vi "NotifyIcon - Create Menu.vi"(8 "error in":errorcluster, 9 "lookup string":string, 11 "Menus":string[][](array[string])=[["item0", "<submenu0>"], ["item1", "submenuitem0"], ["<submenu0>", ""]]) -> (0 "error out":errorcluster, 2 "MenuItem references":refnum<k24>[](array[refnum]))   [LabVIEW 2020]
doc: "Recursive"
uses:
  System.Windows.Forms
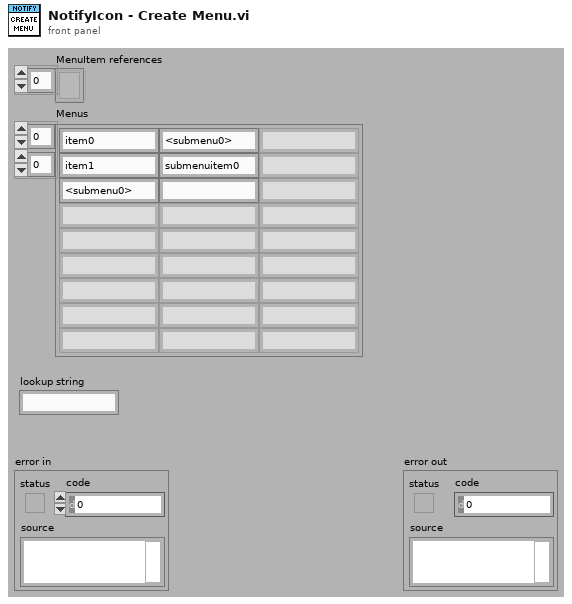
[diagram p1: front panel]
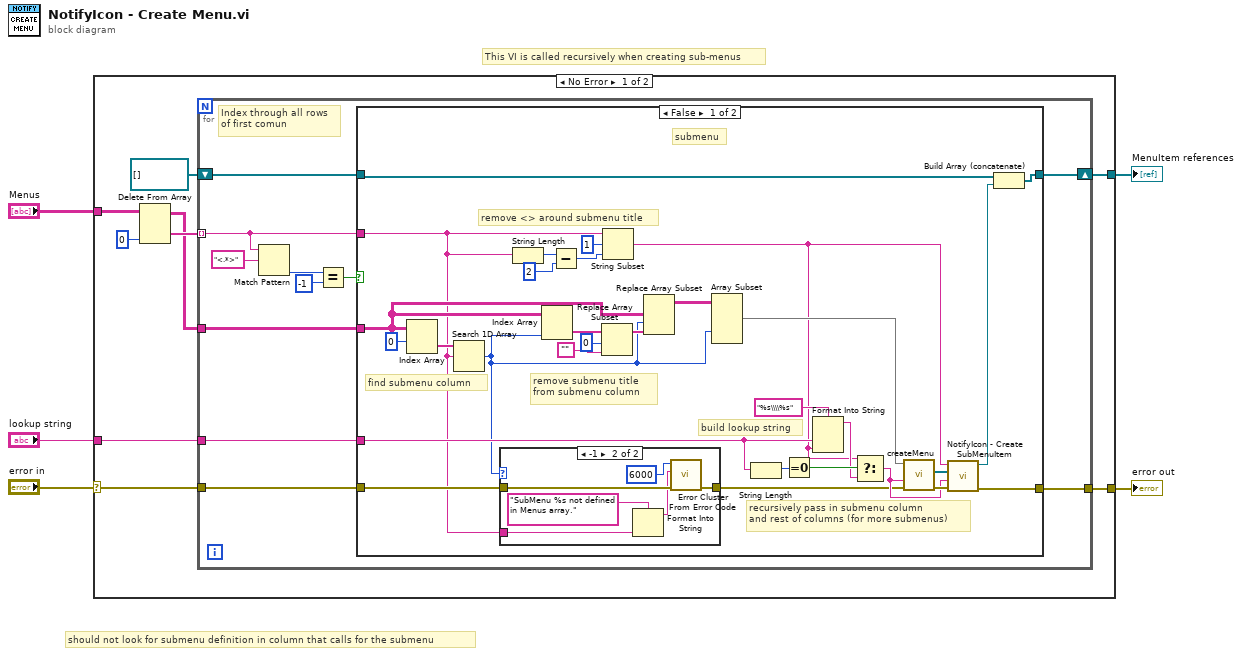
[diagram p0: block diagram]
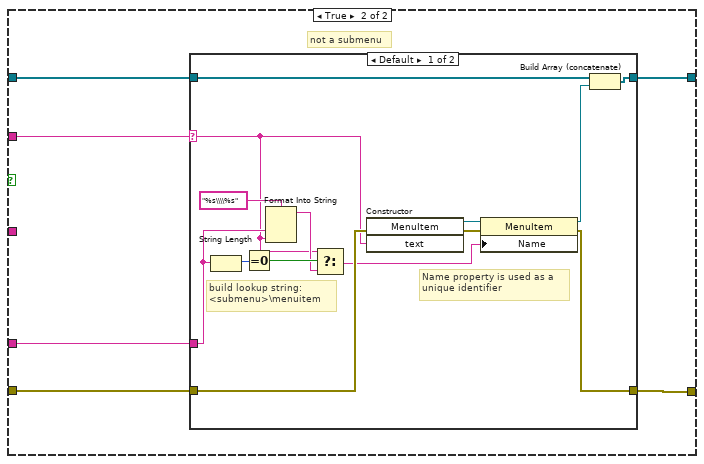
[diagram p3: hidden frame]
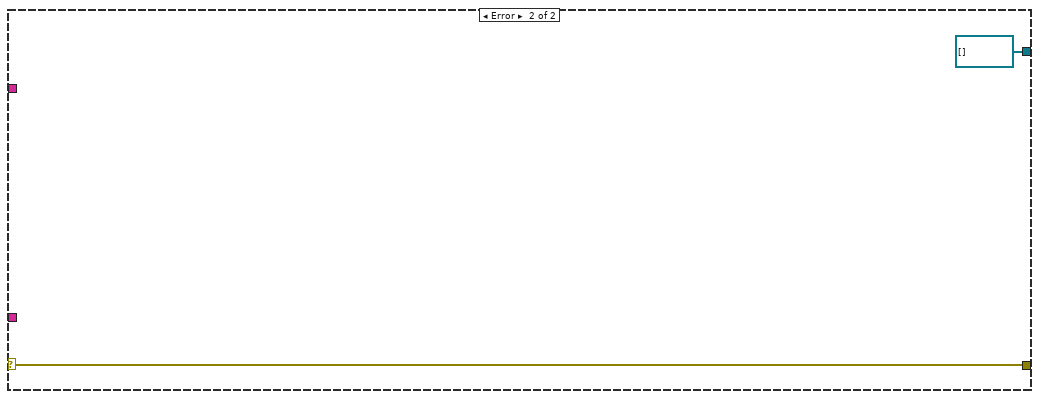
[diagram p5: hidden frame]
diagram:
  # "should not look for submenu definition in column that calls for the submenu"
  # "This VI is called recursively when creating sub-menus"
  n1 = case shown="No Error" "error in" {
    selector: "error in" -> [w10 w86]
    tunnel: [w14 refnum<k24>[] []] -> w5
    tunnel: "Menus" -> [w9 _]
    tunnel: [w12 w86] -> w3
    tunnel: "lookup string" -> [w11 _]
    frame No Error {
      n2 = Delete From Array(array=w9, index (col)=0 ("disabled index (col)")) -> (deleted portion=w7:string[], array with subset deleted=w6:string[][])  [unwired: 2 in]
      n3 = for {
        tunnel: w7 -> [w21] mode=indexing
        shift-right: [w20] -> w14
        shift-left: refnum<k24>[] [] -> [w19]
        tunnel: w6 -> [w18]
        tunnel: w10 -> [w17]
        tunnel: [w16] -> w12
        tunnel: w11 -> [w15]
        # "Index through all rows\nof first comun"
        n4 = Match Pattern(string=w21, regular expression="<.*>") -> (offset past match=w24:i32)  [unwired: 1 in, 3 out]
        n5 = Equal?(x=w24, y=-1) -> (x = y?=w22:bool)
        n6 = case shown="False" w22 {
          tunnel: w21 -> [w26 w64]
          tunnel: [w49 w68] -> w20
          tunnel: w19 -> [w48 w67]
          tunnel: w18 -> [w44 _]
          tunnel: w17 -> [w28 w66]
          tunnel: [w40 w65] -> w16
          tunnel: w15 -> [w35 w63]
          frame False {
            # "build lookup string"
            # "recursively pass in submenu column\nand rest of columns (for more submenus)"
            # "remove submenu title\nfrom submenu column"
            # "find submenu column"
            # "remove <> around submenu title"
            # "submenu"
            n7 = Index Array(array=w44, index (row)=0) -> (element=w50:string[])  [unwired: 1 in]
            n8 = Search 1D Array(1D array=w50, element=w26) -> (index of element=w29:i32)  [unwired: 1 in]
            n9 = case shown="-1" w29 {
              tunnel: w28 -> [w56 w62]
              tunnel: [w56 w61] -> w27
              tunnel: w26 -> [_ w59]
              frame 0, Default {
              }
              frame -1 {
                n10 = Format Into String(format string="SubMenu %s not defined in Menus array." ("error message (\"\")"), w59) -> (resulting string=w58:string)  [unwired: 2 in, 1 out]
                n11 = call <vilib>:"Error Cluster From Error Code.vi"("error in (no error)"=w62, "error message (\"\")"=w58, "error code (0)"=6000) -> ("error out"=w61:errorcluster)  [unwired: 6 in]
              }
            }
            n12 = String Length(string=w26) -> (length=w53:i32)
            n13 = Index Array(array=w44, index (col)=w29) -> (element=w45:string[])  [unwired: 1 in]
            n14 = Subtract(x=w53, y=2) -> (x-y=w51:i32)
            n15 = Replace Array Subset(array=w45, new element="", index=0) -> (w43:string[])
            n16 = String Subset(string=w26, offset (0)=1, length (rest)=w51) -> (substring=w31:string)
            n17 = Replace Array Subset(array=w44, new element=w43, index (col)=w29) -> (w42:string[][])  [unwired: 1 in]
            n18 = Array Subset(array=w42, index (col)=w29) -> (w37:string[][])  [unwired: 3 in]
            n19 = String Length(string=w35) -> (length=w34:i32)
            n20 = Equal To 0?(x=w34) -> (x = 0?=w33:bool)
            n21 = Format Into String(format string="%s\\\\%s", w35, w31) -> (resulting string=w32:string)  [unwired: 2 in, 1 out]
            n22 = Select(t=w31, s=w33, f=w32) -> (s? t:f=w30:string)
            n23 = call "createMenu.vi"("error in"=w27, "lookup string"=w30, "Menus"=w37) -> ("error out"=w39:errorcluster, "MenuItem references"=w46:refnum<k24>[])  [unwired: 7 in]
            n24 = call "NotifyIcon - Create SubMenuItem.vi"("error in"=w39, "lookup string"=w30, "MenuItem references"=w46, "SubMenu Title"=w31) -> ("error out"=w40:errorcluster, "SubMenuItem reference"=w47:refnum<k24>)  [unwired: 6 in]
            n25 = Build Array (concatenate)(w48, w47) -> (w49:refnum<k24>[])
          }
          frame True {
            # "not a submenu"
            n26 = case shown="Default" w64 {
              selector: w64 -> [w70 _]
              tunnel: [w82 w84] -> w68
              tunnel: w67 -> [w81 w84]
              tunnel: w66 -> [w80 w83]
              tunnel: [w77 w83] -> w65
              tunnel: w63 -> [w71 _]
              frame Default {
                # "Name property is used as a \nunique identifier"
                # "build lookup string:\n<submenu>\\menuitem"
                n27 = String Length(string=w71) -> (length=w74:i32)
                n28 = Equal To 0?(x=w74) -> (x = 0?=w73:bool)
                n29 = Format Into String(format string="%s\\\\%s", w71, w70) -> (resulting string=w72:string)  [unwired: 2 in, 1 out]
                n30 = Select(t=w70, s=w73, f=w72) -> (s? t:f=w69:string)
                n31 = constructor class="MenuItem"(error in=w80, "text"=w70) -> (reference out=w79:refnum<k24>, error out=w78:errorcluster)  [unwired: 2 in, 2 out]
                n32 = property class="MenuItem"(reference=w79, error in=w78, "Name"=w69) -> (reference out=w76:refnum<k24>, error out=w77:errorcluster)
                n33 = Build Array (concatenate)(w81, w76) -> (w82:refnum<k24>[])
              }
              frame "" {
                # "skip empty strings\ncreated for 2D array"
              }
            }
          }
        }
      }
    }
    frame Error {
    }
  }
  "MenuItem references" <- w5
  "error out" <- w3
